vi "Relay Control.vi"(8 "error in (no error)":errorcluster, 9 "State":bool, 10 "Channel (0)":u32, 11 "CT Common Tests in":refnum<class "CT Common Tests.lvclass">) -> (0 "error out":errorcluster, 3 "CT Common Tests out":refnum<class "CT Common Tests.lvclass">)   [LabVIEW 2015, in "CT Common Tests.lvclass"]
uses:
  CT Common Tests.lvclass
  Classes/Instruments/Relay Control/Phidget Interface Kit/Class/Phidget Interface Kit 008.lvclass
  Classes/Application/Class/Application.lvclass
  Test Class/Test Class.lvclass
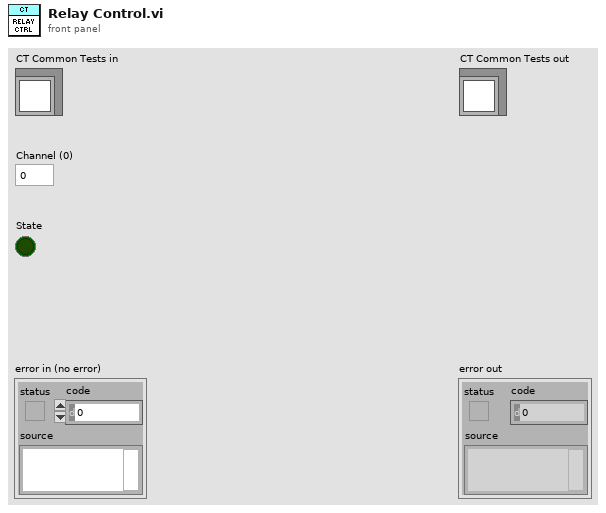
[diagram p1: front panel]
types:
  T1 = typedef "Application.lvlib/App Properties.lvclass/Class Properties -- Cluster.ctl" = cluster{"UUT Info":T2[], "Test Information":refnum<vi>, "Test Complete Event":refnum<user-event>, "Shop Floor System":refnum<class "Shop Floor System.lvclass">, "Gold Board":refnum<class "Golden Board.lvclass">, "Test Recipe":refnum<class "Test Recipe.lvclass">, "Instruments":refnum<class "Instrument.lvclass">[], "Mode":T3, "Test Results":cluster{"Pass":bool[], "Fail Codes":string[]}, "Station Config":refnum<class "Station Config.lvclass">}
  T2 = typedef "Application.lvlib/App Properties.lvclass/UUT Reference -- Cluster.ctl" = cluster{"Serial Number Reference":refnum<vi>, "Status Message Reference":refnum<vi>}
  T3 = typedef "Application.lvlib/Application.lvclass/Op Mode -- Enum.ctl" = u16
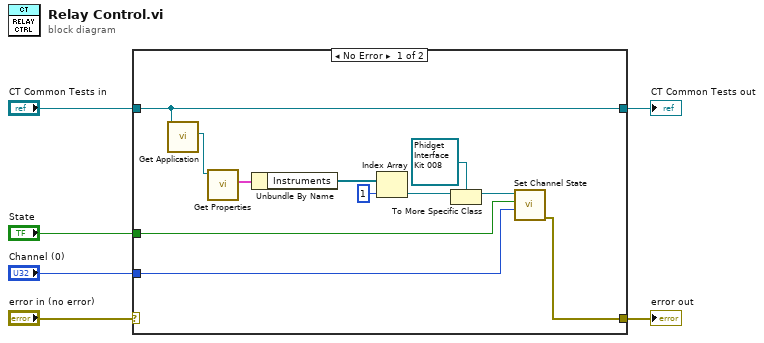
[diagram p0: block diagram]
diagram:
  n1 = case shown="No Error" "error in (no error)" {
    selector: "error in (no error)" -> [_ w19]
    tunnel: [w9 w19] -> w5
    tunnel: [w7 w18] -> w3
    tunnel: "CT Common Tests in" -> [w7 w18]
    tunnel: "Channel (0)" -> [w10 _]
    tunnel: "State" -> [w11 _]
    frame No Error {
      n2 = call "Get Application.vi"("Test Class in"=w7) -> ("Application.lvlib:Application.lvclass"=w16:refnum<class "Application.lvclass">)  [unwired: 9 in, 1 out]
      n3 = call "Get Properties.vi"("Acrobat Template in"=w16) -> ("Class Properties"=w17:T1)  [unwired: 8 in, 2 out]
      n4 = Unbundle By Name(w17) -> ("Instruments"=w8:refnum<class "Instrument.lvclass">[])
      n5 = Index Array(array=w8, index=1) -> (element=w12:refnum<class "Instrument.lvclass">)
      n6 = To More Specific Class(target class=refnum<class "Phidget Interface Kit 008.lvclass"> refnum ("Phidget Interface Kit 008.lvlib:Phidget Interface Kit 008.lvclass"), reference=w12) -> (specific class reference=w15:refnum<class "Phidget Interface Kit 008.lvclass">)  [unwired: 1 in, 1 out]
      n7 = call-dynamic "Set Channel State.vi"("Channel"=w10, "State"=w11, "Acrobat Template in"=w15) -> ("error out"=w9:errorcluster)  [unwired: 7 in, 1 out]
    }
    frame Error {
    }
  }
  "error out" <- w5
  "CT Common Tests out" <- w3
